vi "Init Remote Services.vi"(8 "error in (no error)":errorcluster, 11 "Vecto in":refnum<class "Vecto.lvclass">) -> (0 "error out":errorcluster, 3 "Vecto out":refnum<class "Vecto.lvclass">)   [LabVIEW 2020, in "Vecto.lvlib" / "Vecto.lvclass"]
uses:
  Vecto.lvclass
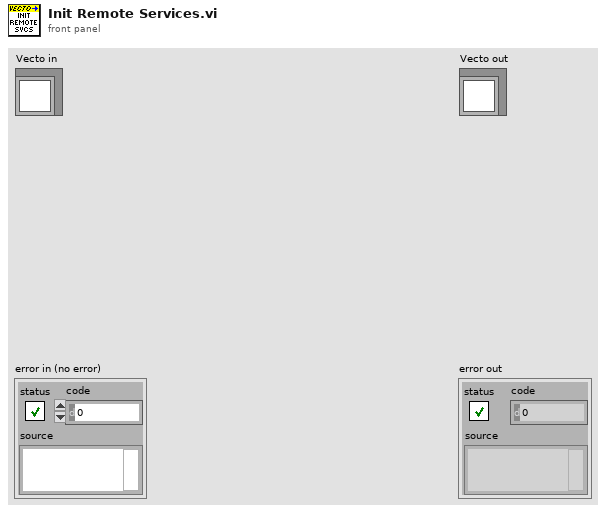
[diagram p1: front panel]
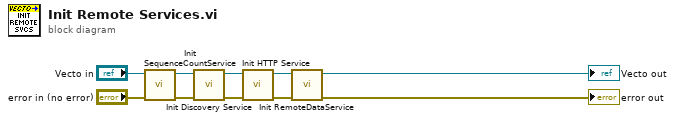
[diagram p0: block diagram]
diagram:
  n1 = call "Init SequenceCountService.vi"("error in (no error)"="error in (no error)", "Vecto in"="Vecto in") -> ("error out"=w8:errorcluster, "Vecto out"=w7:refnum<class "Vecto.lvclass">)  [unwired: 8 in]
  n2 = call "Init Discovery Service.vi"("error in (no error)"=w8, "Vecto in"=w7) -> ("error out"=w9:errorcluster, "Vecto out"=w10:refnum<class "Vecto.lvclass">)  [unwired: 8 in]
  n3 = call "Init HTTP Service.vi"("error in (no error)"=w9, "Vecto in"=w10) -> ("error out"=w6:errorcluster, "Vecto out"=w5:refnum<class "Vecto.lvclass">)  [unwired: 8 in]
  n4 = call "Init RemoteDataService.vi"("error in (no error)"=w6, "Vecto in"=w5) -> ("error out"=→"error out":errorcluster, "Vecto out"=→"Vecto out":refnum<class "Vecto.lvclass">)  [unwired: 8 in]
